vi "Macro Finish Release.vi"(8 "error in (no error)":errorcluster, 11 "Git in":refnum<class "Git.lvclass">) -> (0 "error out":errorcluster, 2 "standard output":string, 3 "Git out":refnum<class "Git.lvclass">)   [LabVIEW 2019, in "Git.lvclass"]
uses:
  Git.lvclass
  Git.lvclass/Git.ctl
  <vilib>/Hampel Software Engineering/Git API/Git API/GIT-api.lvclass
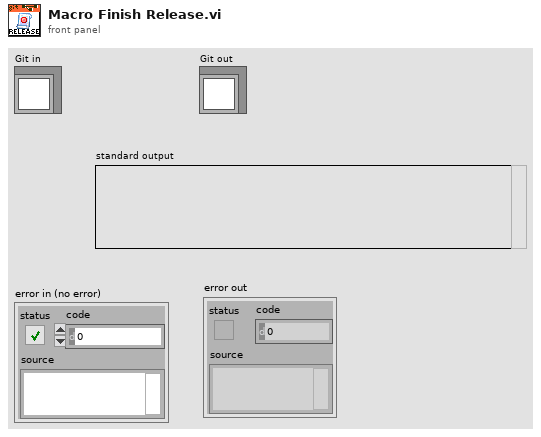
[diagram p1: front panel]
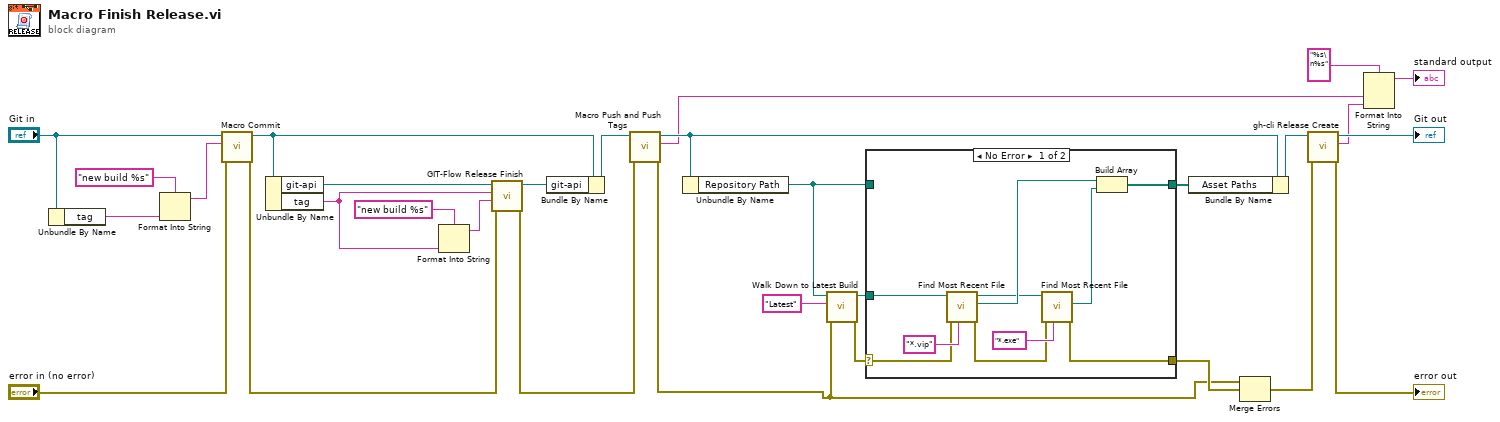
[diagram p0: block diagram]
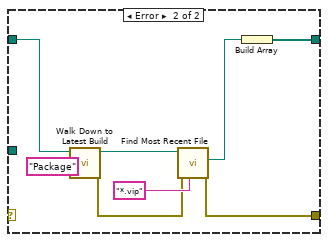
[diagram p2: hidden frame]
diagram:
  n1 = Unbundle By Name("Git in") -> ("tag"=w16:string)
  n2 = Format Into String(format string="new build %s" ("message"), w16) -> (resulting string=w13:string)  [unwired: 2 in, 1 out]
  n3 = call "Macro Commit.vi"("error in (no error)"="error in (no error)", "msg"=w13, "Git in"="Git in") -> ("error out"=w17:errorcluster, "Git out"=w9:refnum<class "Git.lvclass">)  [unwired: 7 in]
  n4 = Unbundle By Name(w9) -> ("git-api"=w20:refnum<class "GIT-api.lvclass">, "tag"=w21:string)
  n5 = Format Into String(format string="new build %s" ("message"), w21) -> (resulting string=w19:string)  [unwired: 2 in, 1 out]
  n6 = call <vilib>:"GIT-Flow Release Finish.vi"("error in"=w17, "message"=w19, "release name"=w21, "Git-API in"=w20) -> ("error out"=w6:errorcluster, "Git-API out"=w8:refnum<class "GIT-api.lvclass">)  [unwired: 6 in]
  n7 = Bundle By Name(cluster=w9, "git-api"=w8) -> (w7:refnum<class "Git.lvclass">)
  n8 = call "Macro Push and Push Tags.vi"("error in (no error)"=w6, "Git in"=w7) -> ("error out"=w1:errorcluster, "std out"=w4:string, "Git out"=w5:refnum<class "Git.lvclass">)  [unwired: 7 in]
  n9 = Unbundle By Name(w5) -> ("Repository Path"=w22:path)
  n10 = call "Walk Down to Latest Build.vi"("error in (no error)"=w1, "name"="Latest", "Repository Path"=w22) -> ("error out"=w23:errorcluster, "Latest Build Folder"=w25:path)  [unwired: 7 in]
  n11 = case shown="No Error" w23 {
    selector: w23 -> [w32 _]
    tunnel: [w40 w48] -> w27
    tunnel: [w39 w46] -> w2
    tunnel: w25 -> [w38 _]
    tunnel: w22 -> [_ w45]
    frame No Error {
      n12 = call "Find Most Recent File.vi"("pattern"="*.vip", "error in (no error)"=w32, "Folder Path"=w38) -> ("error out"=w31:errorcluster, "Newest Path"=w35:path, "dup Folder Path"=w33:path)  [unwired: 6 in]
      n13 = call "Find Most Recent File.vi"("pattern"="*.exe", "error in (no error)"=w31, "Folder Path"=w33) -> ("error out"=w39:errorcluster, "Newest Path"=w34:path)  [unwired: 6 in, 1 out]
      n14 = Build Array(w35, w34) -> (w40:path[])
    }
    frame Error {
      n15 = call "Walk Down to Latest Build.vi"("name"="Package", "Repository Path"=w45) -> ("error out"=w41:errorcluster, "Latest Build Folder"=w43:path)  [unwired: 8 in]
      n16 = call "Find Most Recent File.vi"("pattern"="*.vip", "error in (no error)"=w41, "Folder Path"=w43) -> ("error out"=w46:errorcluster, "Newest Path"=w42:path)  [unwired: 6 in, 1 out]
      n17 = Build Array(w42) -> (w48:path[])
    }
  }
  n18 = Bundle By Name(cluster=w5, "Asset Paths"=w27) -> (w28:refnum<class "Git.lvclass">)
  n19 = Merge Errors(w1, w2) -> (w12:errorcluster)  [unwired: 1 in]
  n20 = call "gh-cli Release Create.vi"("error in (no error)"=w12, "Git in"=w28) -> ("error out"=→"error out":errorcluster, "standard output"=w10:string, "Git out"=→"Git out":refnum<class "Git.lvclass">)  [unwired: 7 in]
  n21 = Format Into String(format string="%s\n%s", w4, w10) -> (resulting string=→"standard output":string)  [unwired: 2 in, 1 out]
